vi "帧同步.vi"() -> ()   [LabVIEW 2010]
uses:
  <vilib>/AddOns/Modulation/Analog/controls/Complex Data Waveform.ctl
  <vilib>/addons/Modulation/Digital/General/MT Generate Bits (Galois, PN Order).vi
  <vilib>/Analysis/2dsp.llb/Real FFT.vi
  <vilib>/imath/engines/lvmath2/RunTimeEngine/ErrorHandling/NIMS_Finalize Error.vi
  <vilib>/imath/engines/lvmath2/RunTimeEngine/RangeToken/NIMS_Range_R2 - Integer.vi
  <instcachedir>/0/NIMS_Range_R2 - Integer_217CA55F27D14E80B3D190635C7B3F47.lvgen/NIMS_Range_R2 - Integer_217CA55F27D14E80B3D190635C7B3F47_000.vi
  <vilib>/imath/engines/lvmath2/RunTimeEngine/NodeEndStatement/NIMS_NodeEndStatement_Output.vi
  <instcachedir>/0/NIMS_NodeEndStatement_Output_53EC0D466D134D7ABD903AC30B43404B.lvgen/NIMS_NodeEndStatement_Output_53EC0D466D134D7ABD903AC30B43404B_004.vi
  <vilib>/imath/engines/lvmath2/RunTimeEngine/CommandStatement/MC_CommandStatement_break.vi
  <vilib>/imath/engines/lvmath2/RunTimeEngine/VariableToken/Read/NIMS_Get Elements - RV(_) - Check.vi
  <instcachedir>/0/NIMS_Get Elements - RV(_) - Check_1F6F8656162345078B1D4DC9877DFAE9.lvgen/NIMS_Get Elements - RV(_) - Check_1F6F8656162345078B1D4DC9877DFAE9_004.vi
  <vilib>/imathl/engines/lvmath/Functions/Error Handling/Create Error.vi
  <vilib>/imath/engines/lvmath2/RunTimeEngine/ReplaceToken/NIMS_Replace - Check Linear.vi
  <instcachedir>/0/NIMS_Replace - Check Linear_662D5651E4E34E0584DA82A256193A4C.lvgen/NIMS_Replace - Check Linear_662D5651E4E34E0584DA82A256193A4C_005.vi
  <vilib>/imath/engines/lvmath2/RunTimeEngine/ReplaceToken/NIMS_Replace - Size Check _(_)=S.vi
  <instcachedir>/0/NIMS_Replace - Size Check _(_)=S_6CAC13ACC74349C582FDAB09BCDAB70F.lvgen/NIMS_Replace - Size Check _(_)=S_6CAC13ACC74349C582FDAB09BCDAB70F_004.vi
  <vilib>/imath/engines/lvmath2/RunTimeEngine/ReplaceToken/NIMS_Replace - V(S)=S.vi
  <instcachedir>/0/NIMS_Replace - V(S)=S_78FDB6CCD265407D8926E4CF958018EB.lvgen/NIMS_Replace - V(S)=S_78FDB6CCD265407D8926E4CF958018EB_002.vi
  <vilib>/imath/engines/lvmath2/RunTimeEngine/BuiltInFunctions/length/NIMS_length(GV).vi
  <instcachedir>/0/NIMS_length(GV)_08A3D13377FD4E4B96F5795FBF3698FA.lvgen/NIMS_length(GV)_08A3D13377FD4E4B96F5795FBF3698FA_001.vi
  <instcachedir>/0/NIMS_NodeEndStatement_Output_53EC0D466D134D7ABD903AC30B43404B.lvgen/NIMS_NodeEndStatement_Output_53EC0D466D134D7ABD903AC30B43404B_009.vi
  <instcachedir>/0/NIMS_NodeEndStatement_Output_53EC0D466D134D7ABD903AC30B43404B.lvgen/NIMS_NodeEndStatement_Output_53EC0D466D134D7ABD903AC30B43404B_008.vi
  <instcachedir>/0/NIMS_NodeEndStatement_Output_53EC0D466D134D7ABD903AC30B43404B.lvgen/NIMS_NodeEndStatement_Output_53EC0D466D134D7ABD903AC30B43404B_000.vi
  <vilib>/imath/engines/lvmath2/RunTimeEngine/BuiltInFunctions/zeros/NIMS_V=zeros(I32,I32).vi
  <instcachedir>/0/NIMS_Replace - Check Linear_662D5651E4E34E0584DA82A256193A4C.lvgen/NIMS_Replace - Check Linear_662D5651E4E34E0584DA82A256193A4C_002.vi
  <instcachedir>/0/NIMS_Get Elements - RV(_) - Check_1F6F8656162345078B1D4DC9877DFAE9.lvgen/NIMS_Get Elements - RV(_) - Check_1F6F8656162345078B1D4DC9877DFAE9_003.vi
  <instcachedir>/0/NIMS_Replace - Size Check _(_)=S_6CAC13ACC74349C582FDAB09BCDAB70F.lvgen/NIMS_Replace - Size Check _(_)=S_6CAC13ACC74349C582FDAB09BCDAB70F_001.vi
  <instcachedir>/0/NIMS_Replace - V(S)=S_78FDB6CCD265407D8926E4CF958018EB.lvgen/NIMS_Replace - V(S)=S_78FDB6CCD265407D8926E4CF958018EB_001.vi
  <vilib>/imath/engines/lvmath2/RunTimeEngine/ErrorHandling/NIMS_Create Error From Enums.vi
  <vilib>/imath/engines/lvmath2/RunTimeEngine/BuiltInFunctions/sum/NIMS_sum(GV).vi
  <instcachedir>/0/NIMS_sum(GV)_67F5EC36BC034E54A6BEC5B0673C00E5.lvgen/NIMS_sum(GV)_67F5EC36BC034E54A6BEC5B0673C00E5_001.vi
  <vilib>/imath/engines/lvmath2/RunTimeEngine/ArithmeticOperatorToken/NIMS_ArithmeticOperator_power(S).vi
  <instcachedir>/0/NIMS_ArithmeticOperator_power(S)_57F73ACEDCCB45A3A88E6DBC6D08A385.lvgen/NIMS_ArithmeticOperator_power(S)_57F73ACEDCCB45A3A88E6DBC6D08A385_010.vi
  <vilib>/imath/engines/lvmath2/RunTimeEngine/BuiltInFunctions/max/1 input/NIMS_max(CV).vi
  <instcachedir>/0/NIMS_max(CV)_76714DD3D95E46BEB090F8BDAA4595CC.lvgen/NIMS_max(CV)_76714DD3D95E46BEB090F8BDAA4595CC_000.vi
  <vilib>/addons/Modulation/niDMT.lvlib
  <vilib>/Analysis/NI_AALPro.lvlib
  <vilib>/addons/Modulation/niAMT.lvlib
panel:
  out "x":cdb
  out "t":i32
  out "dout":dbl[](graph)
  out "FFT {X}":dbl[](graph) caption="FFT{X}"
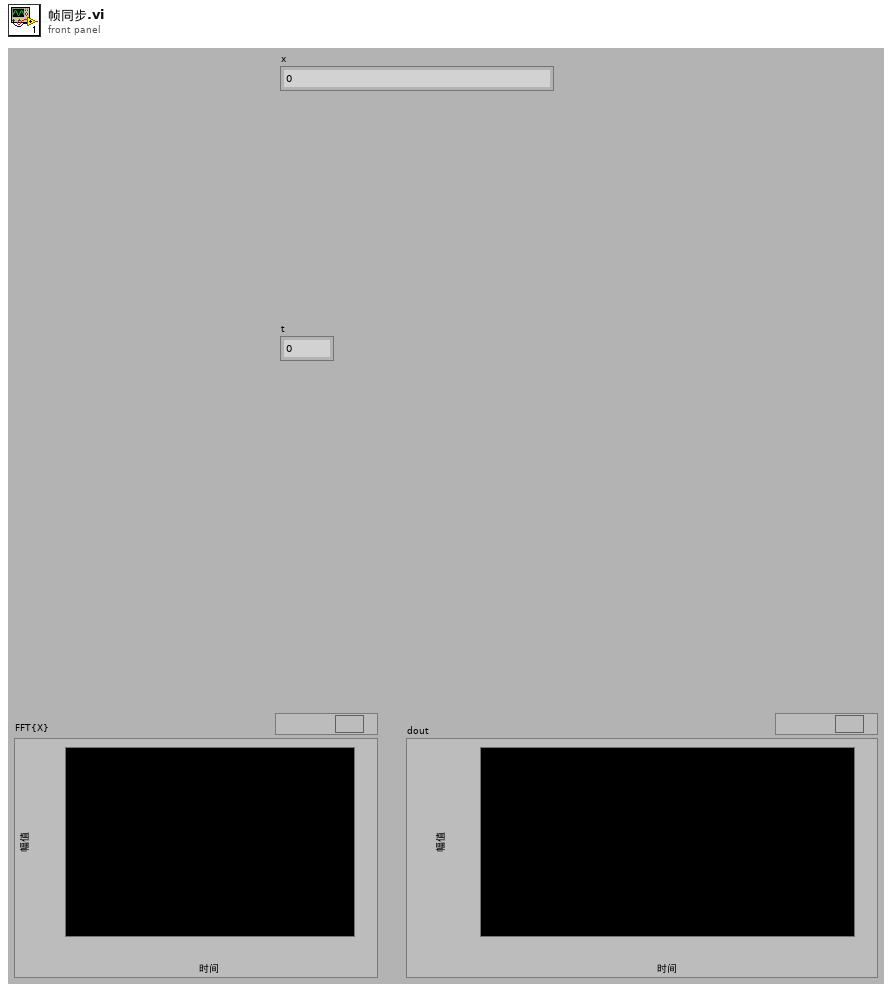
[diagram p1: front panel]
types:
  T1 = typedef "niAMT.lvlib/Complex Data Waveform.ctl" = cluster{"t0":dbl, "dt":dbl, "Y":cdb[]}
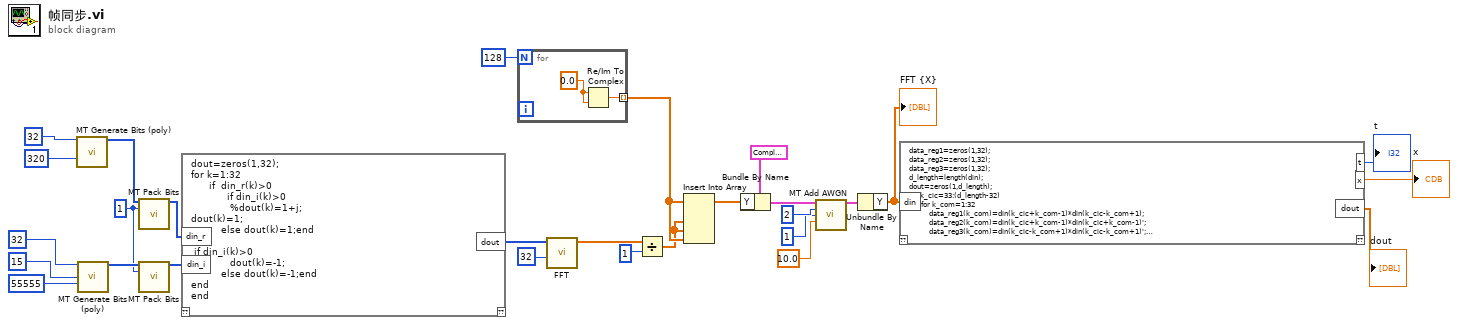
[diagram p0: block diagram]
diagram:
  w21 = 1 ("bits per integer")
  n1 = call-poly <vilib>:"MT Generate Bits (poly).vi"("total bits (128)"=32, "seed in (0xD6BF7DF2)"=320) -> ("output bit stream"=w27:i8[])  [unwired: 11 in, 2 out]
  n2 = call-poly <vilib>:"MT Generate Bits (poly).vi"("total bits (128)"=32, "PN sequence order (9)"=15, "seed in (0xD6BF7DF2)"=55555) -> ("output bit stream"=w23:i8[])  [unwired: 10 in, 2 out]
  n3 = call <vilib>:"MT Pack Bits.vi"("input bit stream"=w27, "bits per integer"=w21) -> ("output integers"=w4:i32[])  [unwired: 12 in, 1 out]
  n4 = call <vilib>:"MT Pack Bits.vi"("input bit stream"=w23, "bits per integer"=w21) -> ("output integers"=w5:i32[])  [unwired: 12 in, 1 out]
  n5 = mathscript code="dout=zeros(1,32);\nfor k=1:32\n      if  din_r(k)>0\n            if din_i(k)>0\n             %dout(k)=1+j;\ndout(k)=1;\n          else dout(k)=1;end\nelse   \n if din_i(k)>0\n             dout(k)=-1;\n          else dout(k)=-1;end\nend\nend"("din_r"=w4, "din_i"=w5) -> ("dout"=w3:i32[])  [unwired: 1 in, 1 out]
  n6 = for {
    N: 128 -> [_]
    tunnel: [w29] -> w10 mode=indexing
    w30 = 0.0
    n7 = Re/Im To Complex(1:w30, 2:w30) -> (0:w29:cdb)
  }
  n8 = call-poly <vilib>:"FFT.vi"("FFT size"=32, "X"=w3) -> ("FFT {X}"=w8:cdb[])  [unwired: 8 in, 1 out]
  n9 = Divide(x=w8, y=1) -> (x/y=w6:cdb[])
  n10 = Insert Into Array(array=w10, new element #1=w6, new element #2=w6, new element #3=w10) -> (w11:cdb[])  [unwired: 1 in]
  n11 = Bundle By Name(cluster=T1 {"t0"=0.0, "dt"=1.0, "Y"=[]} ("input complex waveform"), "Y"=w11) -> (w15:T1)
  n12 = call <vilib>:"MT Add AWGN.vi"("input complex waveform"=w15, "samples per symbol (16)"=2, "bits per symbol (1)"=1, "Eb/N0 (10 dB)"=10.0) -> ("output complex waveform"=w14:T1)  [unwired: 9 in, 2 out]
  n13 = Unbundle By Name(w14) -> ("Y"=w9:cdb[])
  "FFT {X}" <- w9
  n14 = mathscript code="data_reg1=zeros(1,32);\ndata_reg2=zeros(1,32);\ndata_reg3=zeros(1,32);\nd_length=length(din);\ndout=zeros(1,d_length);\nfor k_cic=33:(d_length-32)\n      for k_com=1:32\n          data_reg1(k_com)=din(k_cic+k_com-1)*din(k_cic-k_com+1);\n          data_reg2(k_com)=din(k_cic+k_com-1)*din(k_cic+k_com-1)';\n          data_reg3(k_com)=din(k_cic-k_com+1)*din(k_cic-k_com+1)';\nend\ndout(k_cic)=sum(data_reg1)^2/(sum(data_reg2)*sum(data_reg3));\nend\n%plot(1:d_length,dout);\n[x,t]=max(dout);"("din"=w9) -> ("dout"=→"dout":cdb[], "x"=→"x":cdb, "t"=→"t":i32)  [unwired: 1 in, 1 out]
